vi "FindFirstFreeDiscSpace.vi"(11 "DiscData":i64[](array[numeric])) -> (2 "FreeSpaceFound":bool, 3 "IndexOfFirstFreeDiscSpace":i32)   [LabVIEW 2023, in "2024_9.lvclass"]
uses:
  2024_9.lvclass
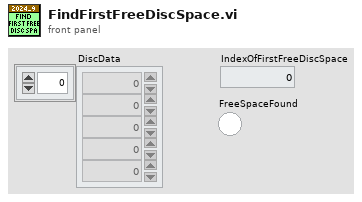
[diagram p1: front panel]
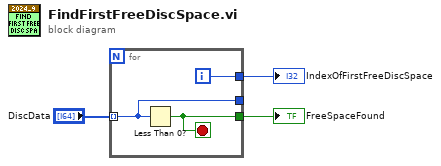
[diagram p0: block diagram]
diagram:
  n1 = for {
    tunnel: "DiscData" -> [w5] mode=indexing
    tunnel: [w6] -> w2
    tunnel: [w5] -> _
    tunnel: [w4] -> w1
    i -> [w6]
    stop <- w4 stop-if-true
    n2 = Less Than 0?(x=w5) -> (x < 0?=w4:bool)
  }
  "IndexOfFirstFreeDiscSpace" <- w2
  "FreeSpaceFound" <- w1
